vi "FFT_DAS-Editing Variables_GBL.vi"() -> ()   [LabVIEW 2018]
doc: "Version: alpha 0.1\nProgrammer: Mike Ashe\n\nGlobal variables for editing the Task Table."
panel:
  in  "Compile Error Index":u32
  out "Compile Errors":cluster{"Line":u32, "Error Message":string}[](array[cluster])
  in  "SearchForError?":bool
  in  "Compile Error Limit":u32=20
  in  "Insert(T)/Overwrite(F)":bool=TRUE
  in  "Block Select":bool
  in  "Block End":i32
  in  "Block Start":i32
  in  "Table Jump":u32=10
  out "Old Edit Pos":cluster{"Row":i32, "Col":i32}
  in  "T-Tbl Clpbd":string[][](table)=[["", "", "", ""], ["", "", "", ""], ["", "", "", ""], ["", "", "", ""], ["", "", "", ""], ["", "", "", ""], ["", "", "", ""], ["", "", "", ""], ["", "", "", ""], ["", "", "", ""]]
  in  "Current Task File":string
  in  "TestTable Changed":bool
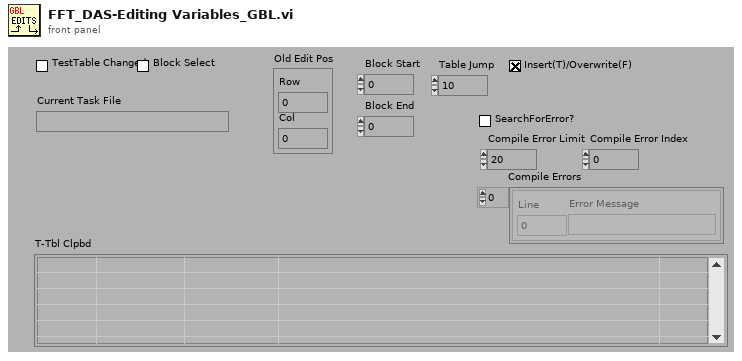
[diagram p1: front panel]
diagram:
